vi "SunplusMTDailyEQC.vi"() -> ()   [LabVIEW 2012]
uses:
  <vilib>/addons/database/Auxilliary.llb/DB Tools Cursor Type.ctl
  <vilib>/Utility/NIReport.llb/NI_report.lvclass
  <vilib>/addons/database/Connection.llb/DB Tools Open Connec (Path).vi
  <vilib>/addons/database/Connection.llb/Conn Execute.vi
  <vilib>/addons/database/Recordset.llb/Rec Fetch Recordset Data (R).vi
  <vilib>/addons/database/Recordset.llb/Rec Destroy - Connection.vi
  <vilib>/addons/database/_DB Variant To Data/Database Variant To Data.xnode
  <vilib>/addons/database/NI_Database_API.lvlib
  <vilib>/Utility/NIReport.llb/Excel/NI_Excel.lvclass
  <vilib>/Utility/SMTP/NI_SMTPEmail.lvlib
panel:
  out "error out 3":errorcluster
  out "concatenated string 2":string
  in  "start (0, 0) 4":cluster{"start row":i32, "start column":i32}
  out "error out 5":errorcluster
  out "concatenated string":string
  out "error out":errorcluster
  out "error out 2":errorcluster
  in  "MIME content-type (application/octet-stream)":string="application/octet-stream"
  out "error out 4":errorcluster
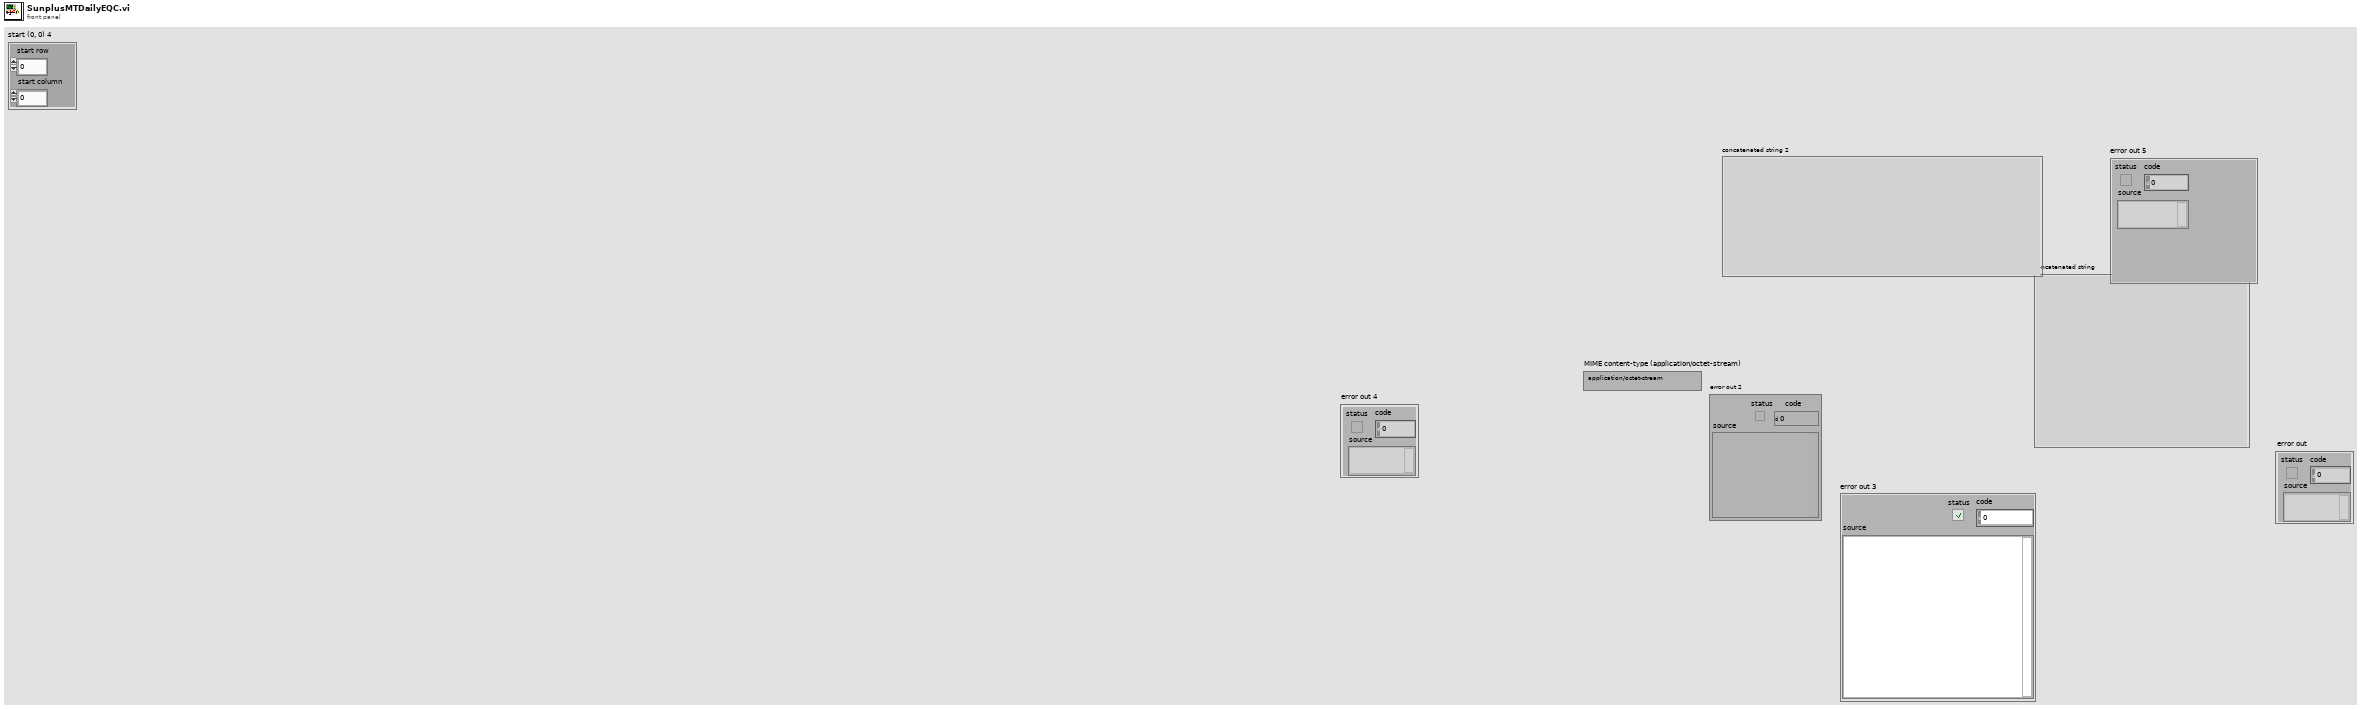
[diagram p1: front panel]
types:
  T1 = typedef "NI_Database_API.lvlib/DB Tools Cursor Type.ctl" = enum16{"forward-only", "keyset", "dynamic", "static"}
  T2 = enum16{"Standard Report", "HTML", "Word", "Excel"}
  T3 = typedef "NI_Database_API.lvlib/Conn ObjectReference.ctl" = refnum<k1>
  T4 = typedef "NI_Database_API.lvlib/Rec ObjectReference.ctl" = refnum<k1>
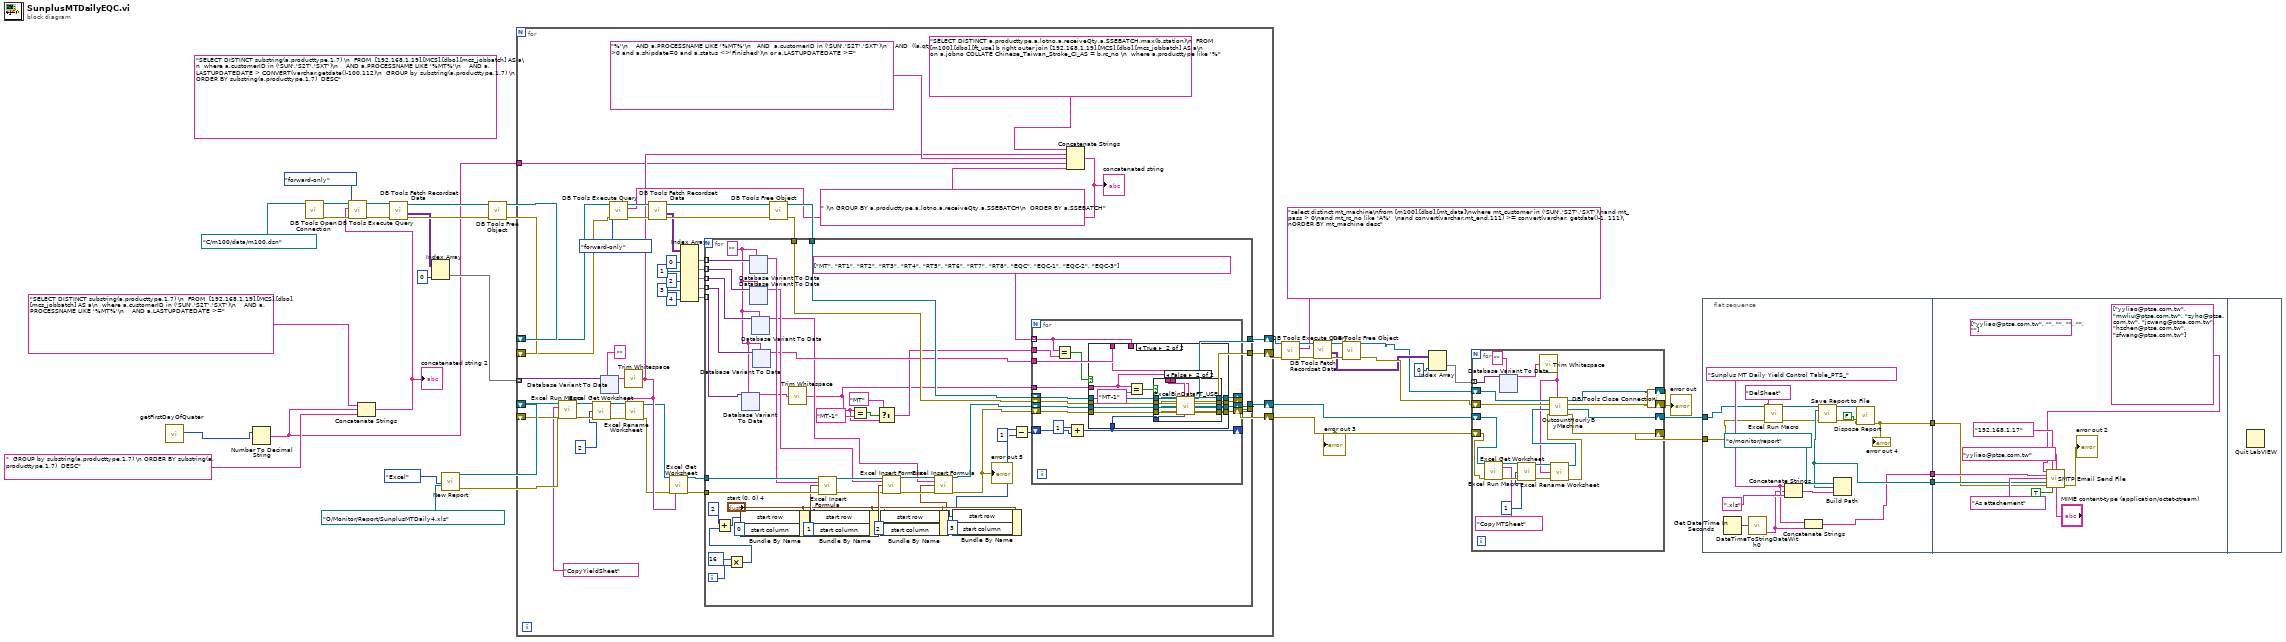
[diagram p0: block diagram]
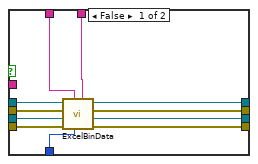
[diagram p2: hidden frame]
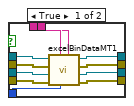
[diagram p3: hidden frame]
diagram:
  (unwired) "SELECT DISTINCT substring(a.producttype,1,7) \n  FROM  [192.168.1.19].[MCS].[dbo].[mcs_jobbatch] AS a\n  where a.customerID in ('SUN','S2T','SXT')\n    AND a.PROCESSNAME LIKE '%MT%'\n    AND a.LASTUPDATEDATE > CONVERT(varchar,getdate()-100,112)\n  GROUP by substring(a.producttype,1,7) \n ORDER BY substring(a.producttype,1,7)  DESC"
  n1 = call "getFirstDayOfQuater.vi"() -> ("FisrtDayofQuater"=w5:i32)  [unwired: 11 in]
  n2 = Number To Decimal String(number=w5) -> (decimal integer string=w1:string)  [unwired: 1 in]
  n3 = call-poly <vilib>:"DB Tools Open Connection.vi"("connection information"=path "C:/m100/data/m100.dsn") -> ("error out"=w28:errorcluster, "connection reference"=w29:T3)  [unwired: 7 in]
  n4 = Concatenate Strings("SELECT DISTINCT substring(a.producttype,1,7) \n  FROM  [192.168.1.19].[MCS].[dbo].[mcs_jobbatch] AS a\n  where a.customerID in ('SUN','S2T','SXT')\n    AND a.PROCESSNAME LIKE '%MT%'\n    AND a.LASTUPDATEDATE >=", w1, "  GROUP by substring(a.producttype,1,7) \n ORDER BY substring(a.producttype,1,7)  DESC") -> (w2:string)
  "concatenated string 2" <- w2
  n5 = call-poly <vilib>:"DB Tools Execute Query.vi"("error in (no error)"=w28, "cursor type"=DB_Tools_Cursor_Type."forward-only", "SQL query"=w2, "connection reference"=w29) -> ("error out"=w26:errorcluster, "recordset reference"=w27:T4)  [unwired: 4 in]
  n6 = call-poly <vilib>:"DB Tools Fetch Recordset Data.vi"("error in (no error)"=w26, "recordset reference"=w27) -> ("error out"=w24:errorcluster, "recordset data"=w18:variant[][], "recordset reference out"=w25:T4)  [unwired: 3 in]
  n7 = Index Array(array=w18, index (col)=0 ("disabled index (col)")) -> (element=w16:variant[])  [unwired: 1 in]
  n8 = call <vilib>:"New Report.vi"("report type"=T2."Excel" ("Report Type"), "template (empty)"=path "O:/Monitor/Report/SunplusMTDaily4.xls") -> ("report out"=w20:refnum<class "NI_report.lvclass">, "error out"=w19:errorcluster)  [unwired: 12 in]
  n9 = call-poly <vilib>:"DB Tools Free Object.vi"("error in (no error)"=w24, "recordset reference"=w25) -> ("error out"=w21:errorcluster, "connection reference"=w22:T3)  [unwired: 8 in]
  n10 = for {
    shift-right: [w86] -> w12
    shift-left: w22 -> [w65]
    shift-right: [w87] -> w11
    shift-left: w21 -> [w64]
    shift-right: [w88] -> w30
    shift-left: w20 -> [w57]
    shift-right: [w89] -> w31
    shift-left: w19 -> [w56]
    tunnel: w16 -> [w63] mode=indexing
    tunnel: w1 -> [w46]
    n11 = call <vilib>:"Excel Run Macro.vi"("report in"=w57, "macro name"="CopyYieldSheet", "error in (no error)"=w56) -> ("report out"=w51:refnum<class "NI_report.lvclass">, "error out"=w50:errorcluster)  [unwired: 10 in, 1 out]
    n12 = call <vilib>:"Excel Get Worksheet.vi"("report in"=w51, "worksheet index (0)"=2, "error in (no error)"=w50) -> ("report out"=w49:refnum<class "NI_report.lvclass">, "error out"=w48:errorcluster)  [unwired: 11 in]
    n13 = xnode "Database Variant To Data"("database variant"=w63, "type"="") -> ("data"=w61:string)  [unwired: 1 in, 1 out]
    n14 = call <vilib>:"Trim Whitespace.vi"("string"=w61) -> ("trimmed string"=w54:string)  [unwired: 1 in]
    n15 = call <vilib>:"Excel Rename Worksheet.vi"("report in"=w49, "worksheet name (\"\")"=w54, "error in (no error)"=w48) -> ("report out"=w53:refnum<class "NI_report.lvclass">, "error out"=w52:errorcluster)  [unwired: 11 in]
    n16 = call <vilib>:"Excel Get Worksheet.vi"("report in"=w53, "error in (no error)"=w52, "name (\"\")"=w54) -> ("report out"=w69:refnum<class "NI_report.lvclass">, "error out"=w68:errorcluster)  [unwired: 11 in]
    n17 = Concatenate Strings("SELECT DISTINCT a.producttype,a.lotno,a.receiveQty,a.SSEBATCH,max(b.station)\n  FROM [m100].[dbo].[ft_use] b right outer join [192.168.1.19].[MCS].[dbo].[mcs_jobbatch] AS a\n  on a.jobno COLLATE Chinese_Taiwan_Stroke_CI_AS = b.rc_no \n  where a.producttype like '%" ("SQL query"), w54, "%'\n    AND a.PROCESSNAME LIKE '%MT%'\n   AND  a.customerID in ('SUN','S2T','SXT')\n    AND  ((a.qty >0 and a.shipdate=0 and a.status <>'Finished')\n or a.LASTUPDATEDATE >=", w46, " )\n GROUP BY a.producttype,a.lotno,a.receiveQty,a.SSEBATCH\n  ORDER BY a.SSEBATCH") -> (w58:string)
    "concatenated string" <- w58
    n18 = call-poly <vilib>:"DB Tools Execute Query.vi"("error in (no error)"=w64, "cursor type"=DB_Tools_Cursor_Type."forward-only", "SQL query"=w58, "connection reference"=w65) -> ("error out"=w82:errorcluster, "recordset reference"=w83:T4)  [unwired: 4 in]
    n19 = call-poly <vilib>:"DB Tools Fetch Recordset Data.vi"("error in (no error)"=w82, "recordset reference"=w83) -> ("error out"=w84:errorcluster, "recordset data"=w80:variant[][], "recordset reference out"=w85:T4)  [unwired: 3 in]
    n20 = Index Array(array=w80, index (col) #1=0 ("disabled index (col)"), index (col) #2=1 ("index (col)"), index (col) #3=2 ("index (col)"), index (col) #4=3 ("index (col)"), index (col) #5=4 ("index (col)")) -> (element #1=w76:variant[], element #2=w75:variant[], element #3=w74:variant[], element #4=w70:variant[], element #5=w66:variant[])  [unwired: 5 in]
    n21 = call-poly <vilib>:"DB Tools Free Object.vi"("error in (no error)"=w84, "recordset reference"=w85) -> ("error out"=w73:errorcluster, "connection reference"=w72:T3)  [unwired: 8 in]
    n22 = for {
      tunnel: w76 -> [w167] mode=indexing
      tunnel: w75 -> [w166] mode=indexing
      tunnel: w74 -> [w165] mode=indexing
      tunnel: w73 -> [w142]
      tunnel: w72 -> [w143]
      tunnel: w70 -> [w164] mode=indexing
      tunnel: w69 -> [w163]
      tunnel: w68 -> [w162]
      tunnel: [w133] -> w88
      tunnel: [w132] -> w89
      tunnel: [w135] -> w86
      tunnel: [w134] -> w87
      tunnel: w66 -> [w129] mode=indexing
      i -> [w146]
      w128 = ""
      n23 = Multiply(x=16, y=w146) -> (x*y=w144:i32)
      n24 = Add(x=2, y=w144) -> (x+y=w139:i32)
      n25 = Bundle By Name(cluster="start (0, 0) 4", "start row"=w139, "start column"=0) -> (w161:cluster{"start row":i32, "start column":i32})
      n26 = xnode "Database Variant To Data"("database variant"=w129, "type"=w128) -> ("data"=w127:string)  [unwired: 1 in, 1 out]
      n27 = xnode "Database Variant To Data"("database variant"=w167, "type"=w128) -> ("data"=w158:string)  [unwired: 1 in, 1 out]
      n28 = xnode "Database Variant To Data"("database variant"=w166, "type"=w128) -> ("data"=w153:string)  [unwired: 1 in, 1 out]
      n29 = xnode "Database Variant To Data"("database variant"=w165, "type"=w128) -> ("data"=w130:string)  [unwired: 1 in, 1 out]
      n30 = xnode "Database Variant To Data"("database variant"=w164, "type"=w128) -> ("data"=w136:string)  [unwired: 1 in, 1 out]
      n31 = call <vilib>:"Trim Whitespace.vi"("string"=w127) -> ("trimmed string"=w122:string)  [unwired: 1 in]
      n32 = Bundle By Name(cluster="start (0, 0) 4", "start row"=w139, "start column"=1) -> (w156:cluster{"start row":i32, "start column":i32})
      n33 = call <vilib>:"Excel Insert Formula.vi"("report in"=w163, "formula"=w158, "start (0, 0)"=w161, "error in (no error)"=w162) -> ("report out"=w155:refnum<class "NI_report.lvclass">, "error out"=w154:errorcluster)  [unwired: 10 in]
      n34 = Equal?(x=w122, y="MT-1") -> (x = y?=w125:bool)
      n35 = Select(t="MT", s=w125, f=w122) -> (s? t:f=w123:string)
      n36 = Bundle By Name(cluster="start (0, 0) 4", "start row"=w139, "start column"=2) -> (w147:cluster{"start row":i32, "start column":i32})
      n37 = call <vilib>:"Excel Insert Formula.vi"("report in"=w155, "formula"=w153, "start (0, 0)"=w156, "error in (no error)"=w154) -> ("report out"=w151:refnum<class "NI_report.lvclass">, "error out"=w150:errorcluster)  [unwired: 10 in]
      n38 = call <vilib>:"Excel Insert Formula.vi"("report in"=w151, "formula"=w130, "start (0, 0)"=w147, "error in (no error)"=w150) -> ("report out"=w141:refnum<class "NI_report.lvclass">, "error out"=w140:errorcluster)  [unwired: 10 in]
      "error out 5" <- w140
      n39 = Bundle By Name(cluster="start (0, 0) 4", "start row"=w139, "start column"=3) -> ()  [unwired: 1 out]
      n40 = Subtract(x=w139, y=1) -> (x-y=w137:i32)
      n41 = for {
        shift-right: [w214] -> w135
        shift-left: w143 -> [w207]
        shift-right: [w213] -> w134
        shift-left: w142 -> [w206]
        shift-right: [w212] -> w133
        shift-left: w141 -> [w205]
        shift-right: [w211] -> w132
        shift-left: w140 -> [w204]
        shift-right: [w210] -> _
        shift-left: w137 -> [w209]
        tunnel: w136 -> [w208]
        tunnel: string[] ["MT", "RT1", "RT2", "RT3", "RT4", "RT5", "RT6", "RT7", "RT8", "EQC", "EQC-1", "EQC-2", "EQC-3"] ("Array") -> [w202] mode=indexing
        tunnel: w123 -> [w203]
        tunnel: w122 -> [w200]
        n42 = Equal?(x=w202, y=w203) -> (x = y?=w201:bool)
        n43 = Add(x=1, y=w209) -> (x+y=w210:i32)
        n44 = case shown="True" w201 {
          tunnel: [w226 w234] -> w214
          tunnel: [w225 w233] -> w213
          tunnel: [w224 w232] -> w212
          tunnel: [w223 w231] -> w211
          tunnel: w210 -> [w222 w239]
          tunnel: w208 -> [w221 w230]
          tunnel: w207 -> [w220 w238]
          tunnel: w206 -> [w219 w237]
          tunnel: w205 -> [w218 w236]
          tunnel: w204 -> [w217 w235]
          tunnel: w202 -> [w216 _]
          tunnel: w200 -> [_ w227]
          frame False {
            n45 = call "ExcelBinData.vi"("step"=w216, "start row"=w222, "jobno"=w221, "error in (no error) 2"=w217, "report in"=w218, "error in (no error)"=w219, "connection reference 2"=w220) -> ("error out 2"=w223:errorcluster, "report out"=w224:refnum<class "NI_report.lvclass">, "error out"=w225:errorcluster, "connection reference"=w226:T3)  [unwired: 1 in]
          }
          frame True {
            n46 = Equal?(x=w227, y="MT-1") -> (x = y?=w228:bool)
            n47 = case shown="False" w228 {
              tunnel: w239 -> [w250 w261]
              tunnel: w238 -> [w249 w260]
              tunnel: w237 -> [w248 w259]
              tunnel: w236 -> [w247 w258]
              tunnel: w235 -> [w246 w257]
              tunnel: [w245 w256] -> w234
              tunnel: [w244 w255] -> w233
              tunnel: [w243 w254] -> w232
              tunnel: [w242 w253] -> w231
              tunnel: w230 -> [w241 w252]
              tunnel: w227 -> [w240 w251]
              frame True {
                n48 = call "excelBinDataMT1.vi"("step"=w240, "start row"=w250, "jobno"=w241, "error in (no error) 2"=w246, "report in"=w247, "error in (no error)"=w248, "connection reference 2"=w249) -> ("error out 2"=w242:errorcluster, "report out"=w243:refnum<class "NI_report.lvclass">, "error out"=w244:errorcluster, "connection reference"=w245:T3)  [unwired: 1 in]
              }
              frame False {
                n49 = call "ExcelBinDataFT_USE.vi"("step"=w251, "start row"=w261, "jobno"=w252, "error in (no error) 2"=w257, "report in"=w258, "error in (no error)"=w259, "connection reference 2"=w260) -> ("error out 2"=w253:errorcluster, "report out"=w254:refnum<class "NI_report.lvclass">, "error out"=w255:errorcluster, "connection reference"=w256:T3)  [unwired: 1 in]
              }
            }
          }
        }
      }
    }
  }
  "error out 3" <- w31
  n50 = call-poly <vilib>:"DB Tools Execute Query.vi"("error in (no error)"=w11, "SQL query"="select distinct mt_machine\nfrom [m100].[dbo].[mt_data]\nwhere mt_customer in ('SUN','S2T','SXT')\nand mt_pass > 0\nand mt_rc_no like 'A%'  \nand convert(varchar,mt_end,111) >= convert(varchar, getdate()-1, 111)\nORDER BY mt_machine desc", "connection reference"=w12) -> ("error out"=w15:errorcluster, "recordset reference"=w14:T4)  [unwired: 5 in]
  n51 = call-poly <vilib>:"DB Tools Fetch Recordset Data.vi"("error in (no error)"=w15, "recordset reference"=w14) -> ("error out"=w13:errorcluster, "recordset data"=w7:variant[][], "recordset reference out"=w10:T4)  [unwired: 3 in]
  n52 = call-poly <vilib>:"DB Tools Free Object.vi"("error in (no error)"=w13, "recordset reference"=w10) -> ("error out"=w8:errorcluster, "connection reference"=w6:T3)  [unwired: 8 in]
  n53 = Index Array(array=w7, index (col)=0 ("disabled index (col)")) -> (element=w38:variant[])  [unwired: 1 in]
  n54 = for {
    tunnel: w38 -> [w409] mode=indexing
    shift-right: [w405] -> w35
    shift-left: w6 -> [w403]
    shift-right: [w404] -> w34
    shift-left: w8 -> [w402]
    shift-right: [w407] -> w33
    shift-left: w30 -> [w395]
    shift-right: [w406] -> w32
    shift-left: w31 -> [w394]
    n55 = call <vilib>:"Excel Run Macro.vi"("report in"=w395, "macro name"="CopyMTSheet", "error in (no error)"=w394) -> ("report out"=w400:refnum<class "NI_report.lvclass">, "error out"=w399:errorcluster)  [unwired: 10 in, 1 out]
    n56 = xnode "Database Variant To Data"("database variant"=w409, "type"="") -> ("data"=w401:string)  [unwired: 1 in, 1 out]
    n57 = call <vilib>:"Excel Get Worksheet.vi"("report in"=w400, "worksheet index (0)"=1, "error in (no error)"=w399) -> ("report out"=w398:refnum<class "NI_report.lvclass">, "error out"=w397:errorcluster)  [unwired: 11 in]
    n58 = call <vilib>:"Trim Whitespace.vi"("string"=w401) -> ("trimmed string"=w391:string)  [unwired: 1 in]
    n59 = call <vilib>:"Excel Rename Worksheet.vi"("report in"=w398, "worksheet name (\"\")"=w391, "error in (no error)"=w397) -> ("report out"=w393:refnum<class "NI_report.lvclass">, "error out"=w392:errorcluster)  [unwired: 11 in]
    n60 = call "OutcountHourlyByMachine.vi"("Machine"=w391, "error in (no error) 2"=w392, "report in"=w393, "error in (no error)"=w402, "connection reference"=w403) -> ("error in (no error) 3"=w406:errorcluster, "report in 2"=w407:refnum<class "NI_report.lvclass">, "error out"=w404:errorcluster, "connection reference 2"=w405:T3)  [unwired: 3 in]
  }
  n61 = call <vilib>:"DB Tools Close Connection.vi"("error in (no error)"=w34, "connection reference"=w35) -> ("error out"=→"error out":errorcluster)  [unwired: 5 in]
  n62 = flat-sequence {
    tunnel: w33 -> [w446]
    tunnel: w32 -> [w444]
    tunnel: [w447] -> w44
    tunnel: [w451] -> w43
    tunnel: [w450] -> w42
    tunnel: w44 -> [w462]
    tunnel: w43 -> [w461]
    tunnel: w42 -> [w460]
    frame #0 {
      w449 = "Sunplus MT Daily Yield Control Table_PTS_" ("string")
      n63 = Get Date/Time In Seconds() -> (seconds since 1Jan1904=w453:timestamp)
      n64 = call "DateTimeToStringDateWith0.vi"("time stamp"=w453) -> ("Dateyyyymmdd"=w448:string)  [unwired: 9 in, 1 out]
      n65 = call <vilib>:"Excel Run Macro.vi"("report in"=w446, "macro name"="DelSheet", "error in (no error)"=w444) -> ("report out"=w445:refnum<class "NI_report.lvclass">, "error out"=w443:errorcluster)  [unwired: 10 in, 1 out]
      n66 = Concatenate Strings(w449, w448, ".xls" ("string")) -> (w452:string)
      n67 = Concatenate Strings(w449, w448) -> (w447:string)
      n68 = Build Path(base path=path "o:/monitor/report", name or relative path=w452) -> (appended path=w451:path)
      n69 = call-dynamic "Save Report to File.vi"("report in"=w445, "report file path"=w451, "error in (no error)"=w443) -> ("report out"=w456:refnum<class "NI_report.lvclass">, "error out"=w455:errorcluster)  [unwired: 11 in]
      n70 = call-dynamic "Dispose Report.vi"("report in"=w456, "save changes? (F)"=FALSE, "error in (no error)"=w455) -> ("error out"=w450:errorcluster)  [unwired: 12 in]
      "error out 4" <- w450
    }
    frame #1 {
      (unwired) string[] ["yyliao@ptse.com.tw", "", "", "", "", ""] ("recipients")
      n71 = call <vilib>:"SMTP Email Send File.vi"("recipients"=string[] ["yyliao@ptse.com.tw", "mwliu@ptse.com.tw", "zyho@ptse.com.tw", "jcwang@ptse.com.tw", "hzchen@ptse.com.tw", "sfwang@ptse.com.tw"], "mail server"="192.168.1.17", "return address"="yyliao@ptse.com.tw", "subject ([No Subject])"=w462, "message"="As attachement", "file path"=w461, "error in (no error)"=w460, "binary? (F)"=TRUE, "MIME content-type (application/octet-stream)"="MIME content-type (application/octet-stream)") -> ("error out"=→"error out 2":errorcluster)  [unwired: 5 in, 1 out]
    }
    frame #2 {
      n72 = Quit LabVIEW() -> ()  [unwired: 1 in]
    }
  }
